vi "IIR LP I32.vi"(7 "Reset":bool=TRUE, 8 "input valid":bool=TRUE, 9 "b0":fxp<+/-,32,2>, 10 "a0":fxp<+/-,32,2>, 11 "Value in":fxp<+/-,32,14>) -> (0 "output valid":bool, 3 "Value out":fxp<+/-,32,14>)   [LabVIEW 2018]
doc: "Calculates\ny(n) = a0*x(n) + b0*y(n-1)\nwhere y is output signal, x is input"
uses:
  <vilib>/rvi/FXPMathLib/FxpConvert/subVIs/nifxpmath_Convert_SimConfig.ctl
  <vilib>/fxp/LVFixedPointQuantizationPolicyTypeDef.ctl
  <vilib>/fxp/LVFixedPointOverflowPolicyTypeDef.ctl
  <vilib>/rvi/FXPMathLib/FxpConvert/simVIs/DllFxpConvertTemp_sub.vi
  <vilib>/rvi/FXPMathLib/FxpAdd/XNode/nifxpmath_Add.xnode
  <vilib>/rvi/FXPMathLib/FxpConvert/XNode/nifxpmath_Convert.xnode
  <vilib>/rvi/FXPMathLib/FxpMul/XNode/nifxpmath_Multiplier.xnode
  <vilib>/rvi/FXPMathLib/sim/FxpSim.dll
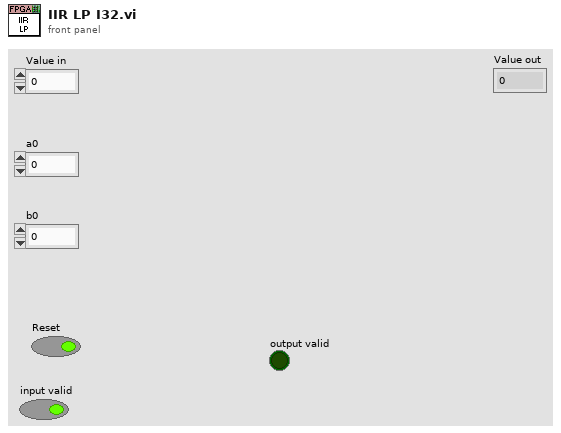
[diagram p1: front panel]
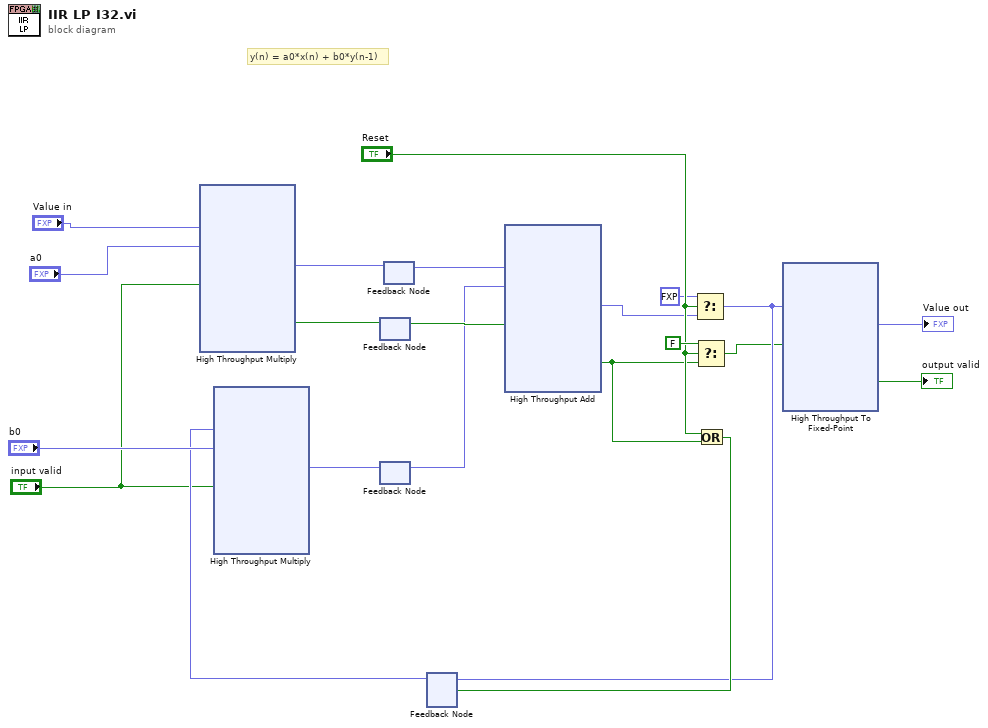
[diagram p0: block diagram]
diagram:
  # "y(n) = a0*x(n) + b0*y(n-1)"
  n1 = xnode ("High Throughput Multiply")("x"="Value in", "y"="a0", "input valid"="input valid") -> ("x*y"=w18:fxp<+/-,32,21>, "output valid"=w17:bool)  [unwired: 1 in, 1 out]
  n2 = feedback #1() -> (w14:bool)  [unwired: 1 in]
  n3 = feedback-in #1(w17) -> ()
  n4 = feedback #2() -> (w13:fxp<+/-,32,21>)  [unwired: 1 in]
  n5 = feedback-in #3(w18) -> ()
  n6 = feedback #3() -> (w15:fxp<+/-,32,21>)  [unwired: 1 in]
  n7 = feedback #4() -> (w12:fxp<+/-,32,21>)  [unwired: 1 in]
  n8 = xnode ("High Throughput Multiply")("x"=w12, "y"="b0", "input valid"="input valid") -> ("x*y"=w16:fxp<+/-,32,21>)  [unwired: 1 in, 2 out]
  n9 = feedback-in #2(w16) -> ()
  n10 = xnode ("High Throughput Add")("x"=w15, "y"=w13, "input valid"=w14) -> ("x+y"=w6:fxp<+/-,32,21>, "output valid"=w5:bool)  [unwired: 1 in, 1 out]
  n11 = Select(t=fxp<+/-,32,21> 0.0, s="Reset", f=w6) -> (s? t:f=w7:fxp<+/-,32,21>)
  n12 = Select(t=FALSE, s="Reset", f=w5) -> (s? t:f=w3:bool)
  n13 = Or(x="Reset", y=w5) -> (x .or. y?=w8:bool)
  n14 = feedback-in #4(w7, w8) -> ()
  n15 = xnode "High Throughput To Fixed-Point"("x"=w7, "input valid"=w3) -> ("y"=→"Value out":fxp<+/-,32,14>, "output valid"=→"output valid":bool)  [unwired: 1 in, 1 out]
